vi "(SubVI) Calculate WLC Fit Curve.vi"(5 "Enum 2":T1(ring), 6 "Force Upper Limit":dbl=10.0, 7 "OneSide? \n(only >0)":bool=TRUE, 8 "BestFit":dbl[](array[numeric])=[45.0, 1150.0]) -> (1 "Fit Force (pN)":dbl[](array[numeric]), 3 "Fit Extension (nm)":dbl[](array[numeric]))   [LabVIEW 2014]
panel:
  out "x-y":dbl
  out "output variable":dbl
  in  "input variable":dbl
  out "size(s) 2":i32
  out "size(s)":i32
  out "Force (pN)":dbl[](array[numeric])
  out "XY Graph":cluster{dbl[], dbl[]}(graph)
  out "dF (pN)":dbl
  out "dL (nm) or K (pN)":dbl
  out "Lc (nm)":dbl
  out "Lp (nm)":dbl
  out "Extension (nm)":dbl[](array[numeric])
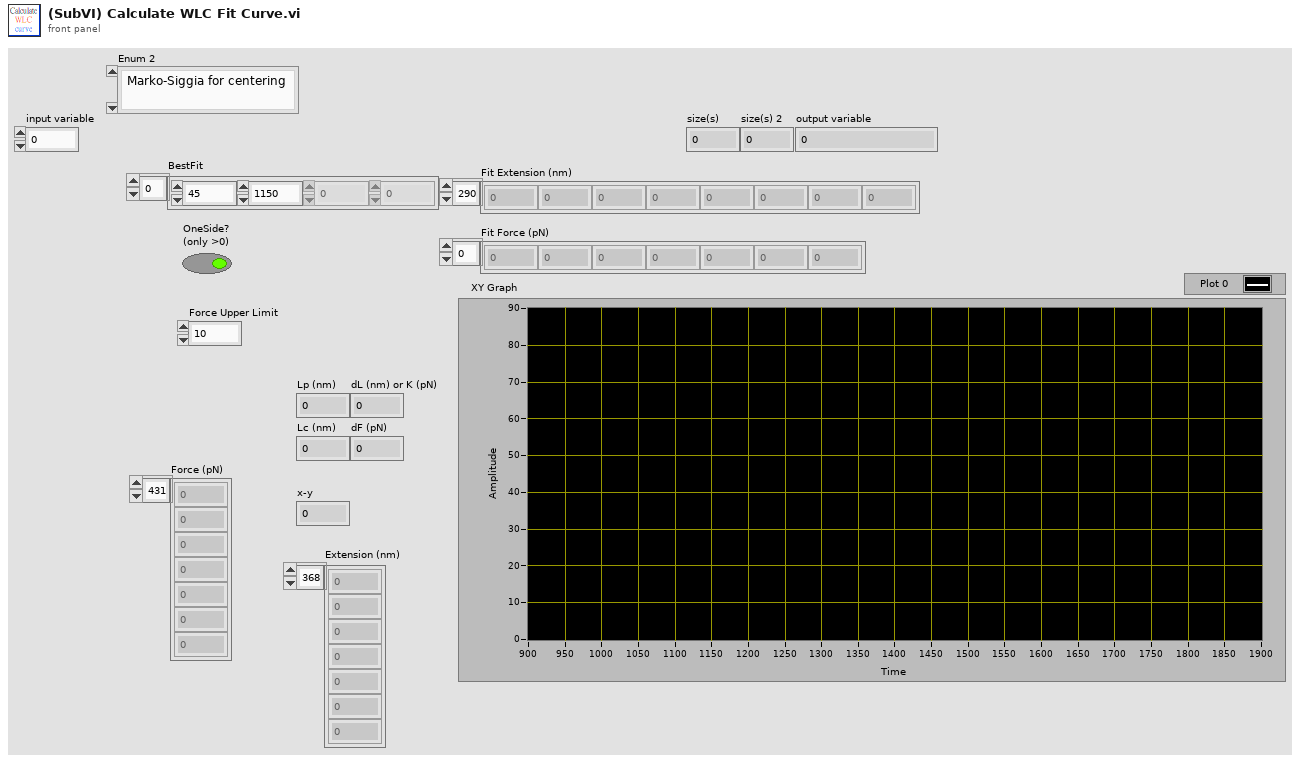
[diagram p1: front panel]
types:
  T1 = enum16{" Marko-Siggia for centering", "Marko-Siggia", "direct fit (Lp,Lc,K)", "fit K (Lp,Lc,K)", "eWLC (Lp=45,Lc,K)"}
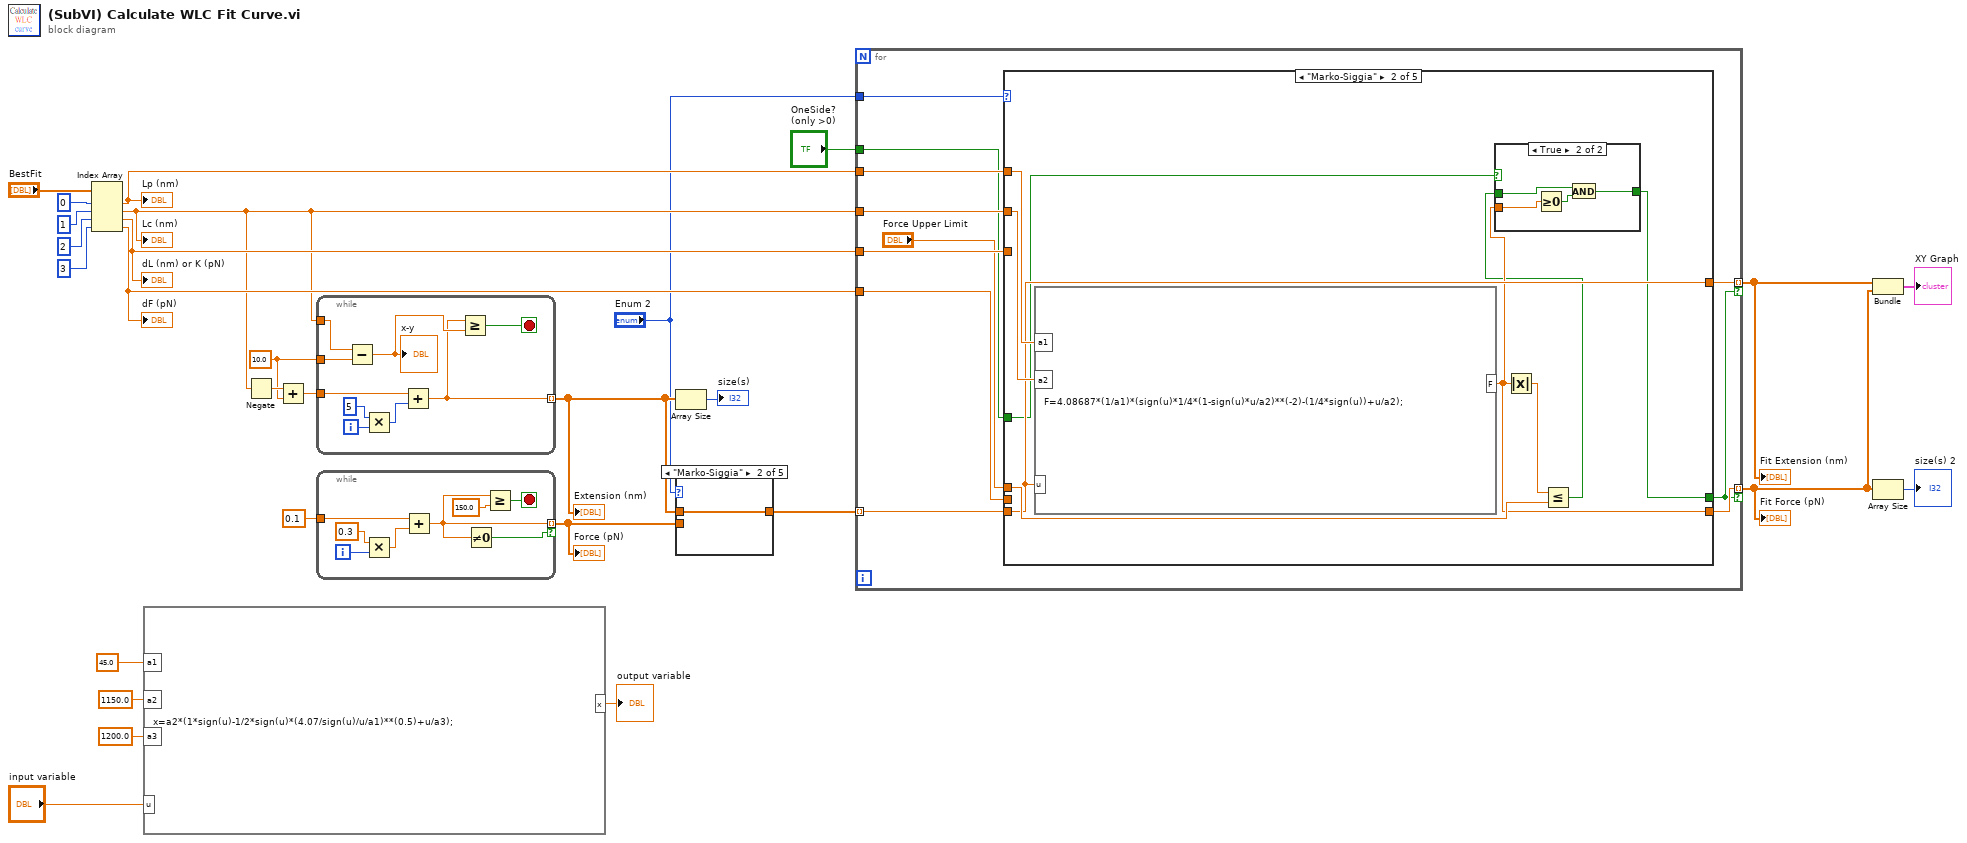
[diagram p0: block diagram]
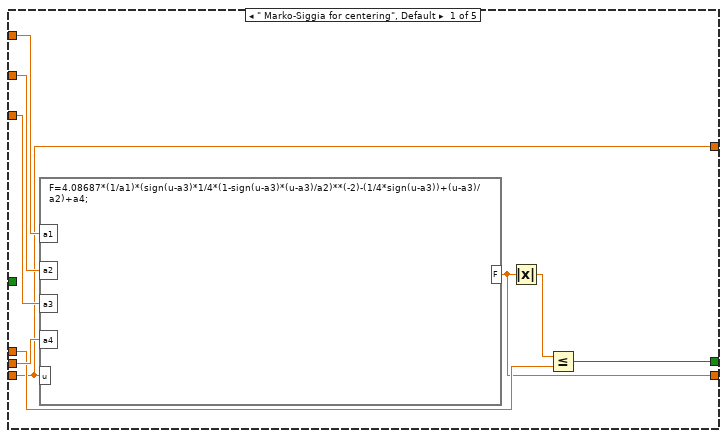
[diagram p6: hidden frame]
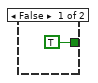
[diagram p7: hidden frame]
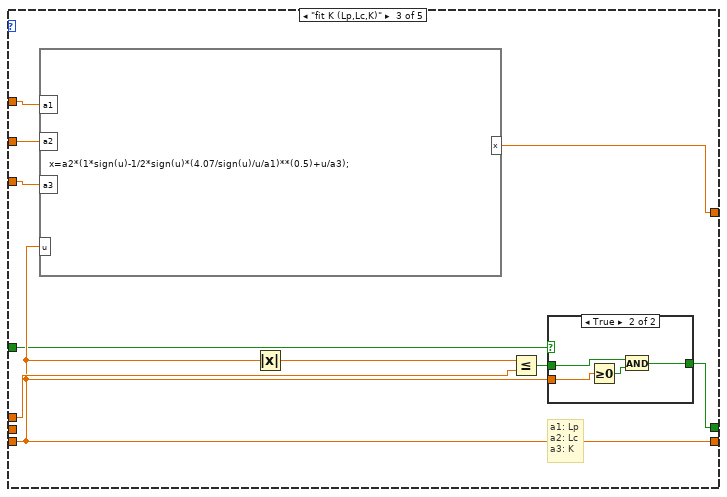
[diagram p8: hidden frame]
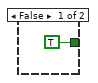
[diagram p9: hidden frame]
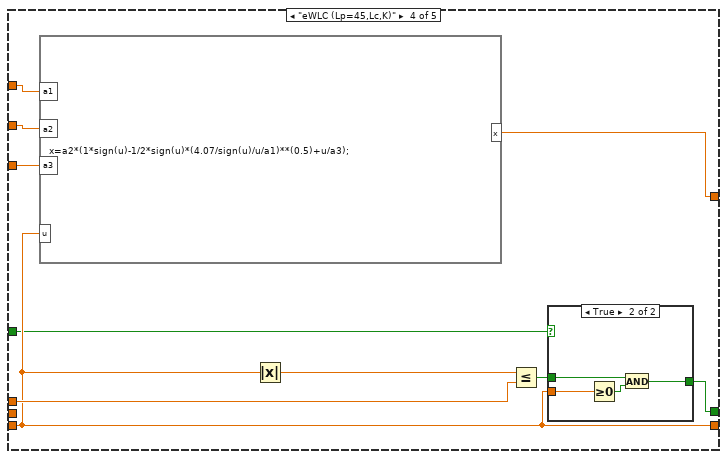
[diagram p10: hidden frame]
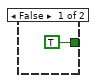
[diagram p11: hidden frame]
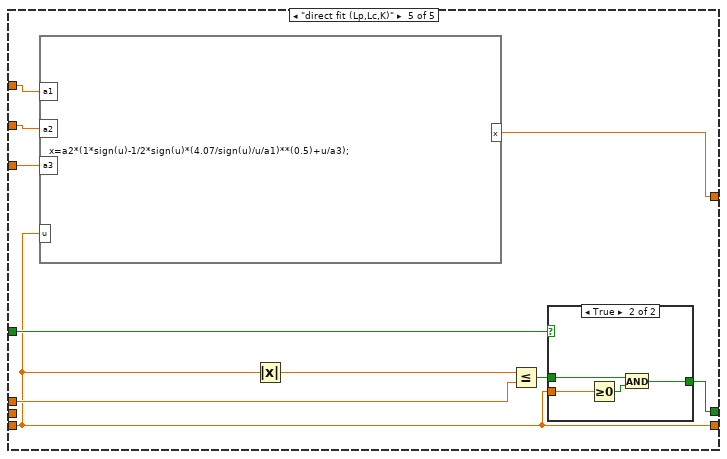
[diagram p12: hidden frame]
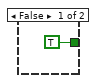
[diagram p13: hidden frame]
diagram:
  w16 = 10.0
  n1 = Index Array(array="BestFit", index #1=0 ("index"), index #2=1 ("index"), index #3=2 ("index"), index #4=3 ("index")) -> (element #1=w23:dbl, element #2=w19:dbl, element #3=w22:dbl, element #4=w21:dbl)
  "Lp (nm)" <- w23
  "Lc (nm)" <- w19
  "dL (nm) or K (pN)" <- w22
  "dF (pN)" <- w21
  n2 = formula code="x=a2*(1*sign(u)-1/2*sign(u)*(4.07/sign(u)/u/a1)**(0.5)+u/a3);"("a1"=45.0 ("input variable"), "a2"=1150.0 ("input variable"), "u"="input variable", "a3"=1200.0 ("input variable")) -> ("x"=→"output variable":dbl)
  n3 = Negate(x=w19) -> (-x=w18:dbl)
  n4 = Add(x=w18, y=w16) -> (x+y=w17:dbl)
  n5 = while {
    tunnel: w19 -> [w34]
    tunnel: [w31] -> w11 mode=indexing
    tunnel: w17 -> [w30]
    tunnel: w16 -> [w29]
    i -> [w37]
    stop <- w32 stop-if-true
    n6 = Subtract(x=w34, y=w29) -> (x-y=w33:dbl)
    "x-y" <- w33
    n7 = Multiply(x=5, y=w37) -> (x*y=w35:i32)
    n8 = Add(x=w30, y=w35) -> (x+y=w31:dbl)
    n9 = Greater Or Equal?(x=w31, y=w33) -> (x >= y?=w32:bool)
  }
  "Extension (nm)" <- w11
  n10 = while {
    tunnel: 0.1 ("y") -> [w43]
    tunnel: [w39] -> w10 mode=indexing if=w38
    i -> [w45]
    stop <- w42 stop-if-true
    n11 = Multiply(x=0.3, y=w45) -> (x*y=w44:dbl)
    n12 = Add(x=w43, y=w44) -> (x+y=w39:dbl)
    n13 = Not Equal To 0?(x=w39) -> (x != 0?=w38:bool)
    n14 = Greater Or Equal?(x=w39, y=150.0) -> (x >= y?=w42:bool)
  }
  "Force (pN)" <- w10
  n15 = Array Size(array=w11) -> (size(s)=→"size(s)":i32)
  n16 = case shown="\"Marko-Siggia\"" "Enum 2" {
    tunnel: w11 -> [w46 w47 _ _ _]
    tunnel: [w46 w47 w48 w49 w50] -> w9
    tunnel: w10 -> [_ _ w48 w49 w50]
    frame " Marko-Siggia for centering", Default {
    }
    frame "Marko-Siggia" {
    }
    frame "fit K (Lp,Lc,K)" {
    }
    frame "eWLC (Lp=45,Lc,K)" {
    }
    frame "direct fit (Lp,Lc,K)" {
    }
  }
  n17 = for {
    tunnel: w23 -> [w61]
    tunnel: w19 -> [w60]
    tunnel: w22 -> [w59]
    tunnel: w21 -> [w58]
    tunnel: w9 -> [w57] mode=indexing
    tunnel: [w54] -> w12 mode=indexing if=w52
    tunnel: [w53] -> w15 mode=indexing if=w52
    tunnel: "Enum 2" -> [w56]
    tunnel: "OneSide? \n(only >0)" -> [w51]
    n18 = case shown="\"Marko-Siggia\"" w56 {
      tunnel: w61 -> [w70 w79 w91 w109 w123]
      tunnel: w60 -> [w69 w78 w90 w108 w122]
      tunnel: w59 -> [w68 _ w94 w105 w124]
      tunnel: w58 -> [w67 _ _ _ _]
      tunnel: w57 -> [w64 w76 w86 w103 w117]
      tunnel: [w63 w74 w86 w103 w117] -> w54
      tunnel: [w65 w71 w87 w101 w115] -> w52
      tunnel: "Force Upper Limit" -> [w66 w77 w93 w107 w119]
      tunnel: [w64 w76 w92 w106 w121] -> w53
      tunnel: w51 -> [_ w73 w85 w100 w118]
      frame " Marko-Siggia for centering", Default {
        n19 = formula code="F=4.08687*(1/a1)*(sign(u-a3)*1/4*(1-sign(u-a3)*(u-a3)/a2)**(-2)-(1/4*sign(u-a3))+(u-a3)/a2)+a4;"("a1"=w70, "a2"=w69, "a3"=w68, "a4"=w67, "u"=w64) -> ("F"=w63:dbl)
        n20 = Absolute Value(x=w63) -> (abs(x)=w62:dbl)
        n21 = Less Or Equal?(x=w62, y=w66) -> (x <= y?=w65:bool)
      }
      frame "Marko-Siggia" {
        n22 = formula code="F=4.08687*(1/a1)*(sign(u)*1/4*(1-sign(u)*u/a2)**(-2)-(1/4*sign(u))+u/a2);"("a1"=w79, "a2"=w78, "u"=w76) -> ("F"=w74:dbl)
        n23 = Absolute Value(x=w74) -> (abs(x)=w75:dbl)
        n24 = Less Or Equal?(x=w75, y=w77) -> (x <= y?=w72:bool)
        n25 = case shown="True" w73 {
          tunnel: w72 -> [_ w83]
          tunnel: [TRUE w82] -> w71
          tunnel: w74 -> [_ w81]
          frame False {
          }
          frame True {
            n26 = Greater Or Equal To 0?(x=w81) -> (x >= 0?=w84:bool)
            n27 = And(x=w83, y=w84) -> (x .and. y?=w82:bool)
          }
        }
      }
      frame "fit K (Lp,Lc,K)" {
        # "a1: Lp\na2: Lc\na3: K"
        n28 = formula code="x=a2*(1*sign(u)-1/2*sign(u)*(4.07/sign(u)/u/a1)**(0.5)+u/a3);"("a1"=w91, "a2"=w90, "u"=w86, "a3"=w94) -> ("x"=w92:dbl)
        n29 = Absolute Value(x=w86) -> (abs(x)=w89:dbl)
        n30 = Less Or Equal?(x=w89, y=w93) -> (x <= y?=w88:bool)
        n31 = case shown="True" w85 {
          tunnel: w88 -> [_ w98]
          tunnel: [TRUE w97] -> w87
          tunnel: w86 -> [_ w96]
          frame False {
          }
          frame True {
            n32 = Greater Or Equal To 0?(x=w96) -> (x >= 0?=w99:bool)
            n33 = And(x=w98, y=w99) -> (x .and. y?=w97:bool)
          }
        }
      }
      frame "eWLC (Lp=45,Lc,K)" {
        n34 = formula code="x=a2*(1*sign(u)-1/2*sign(u)*(4.07/sign(u)/u/a1)**(0.5)+u/a3);"("a1"=w109, "a2"=w108, "u"=w103, "a3"=w105) -> ("x"=w106:dbl)
        n35 = Absolute Value(x=w103) -> (abs(x)=w104:dbl)
        n36 = Less Or Equal?(x=w104, y=w107) -> (x <= y?=w102:bool)
        n37 = case shown="True" w100 {
          tunnel: w103 -> [_ w113]
          tunnel: w102 -> [_ w112]
          tunnel: [TRUE w111] -> w101
          frame False {
          }
          frame True {
            n38 = Greater Or Equal To 0?(x=w113) -> (x >= 0?=w114:bool)
            n39 = And(x=w112, y=w114) -> (x .and. y?=w111:bool)
          }
        }
      }
      frame "direct fit (Lp,Lc,K)" {
        n40 = formula code="x=a2*(1*sign(u)-1/2*sign(u)*(4.07/sign(u)/u/a1)**(0.5)+u/a3);"("a1"=w123, "a2"=w122, "u"=w117, "a3"=w124) -> ("x"=w121:dbl)
        n41 = Absolute Value(x=w117) -> (abs(x)=w120:dbl)
        n42 = Less Or Equal?(x=w120, y=w119) -> (x <= y?=w116:bool)
        n43 = case shown="True" w118 {
          tunnel: w117 -> [_ w128]
          tunnel: w116 -> [_ w127]
          tunnel: [TRUE w126] -> w115
          frame False {
          }
          frame True {
            n44 = Greater Or Equal To 0?(x=w128) -> (x >= 0?=w129:bool)
            n45 = And(x=w127, y=w129) -> (x .and. y?=w126:bool)
          }
        }
      }
    }
  }
  "Fit Force (pN)" <- w12
  "Fit Extension (nm)" <- w15
  n46 = Bundle(w15, w12) -> (→"XY Graph":cluster{dbl[], dbl[]})  [unwired: 1 in]
  n47 = Array Size(array=w12) -> (size(s)=→"size(s) 2":i32)
